vi "Check ref frame selected (simple).vi"() -> (3 "Proceed / Ref frame ok":bool)   [LabVIEW 2020]
uses:
  Typedefs/Set Main VI cursor.ctl
  Global Variables/General Globals.vi
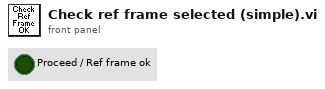
[diagram p1: front panel]
types:
  T1 = typedef "Set Main VI cursor.ctl" = enum16{"Release busy cursor", "Set busy cursor"}
  T2 = typedef "Reference_Globals.ctl" = cluster{"Refrence data path":path, "Reference Rectangle":i16[][], "AOL Z":dbl, "No of pixels in a miniscan ":i32[], "Threshold":i16[], "No of miniscans":i32[], "Full Frame Size":u16, "Reference Image":T3, "dwelltime":dbl, "Zoom":dbl, "Field of View":dbl, "Z Step":i8, "Z pixels":i32, "Z Lines":u8, "Z Ignore":u8, "Laser":u8}
  T3 = typedef "IMAQ Image.ctl" = refnum<image>
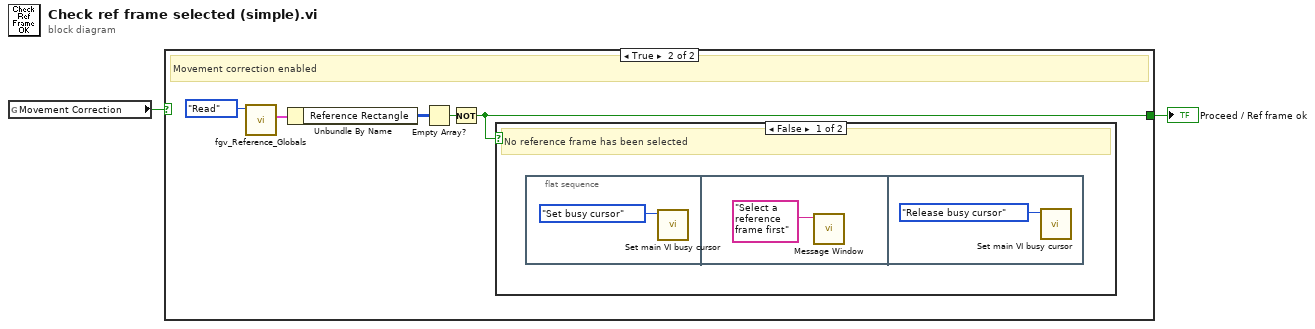
[diagram p0: block diagram]
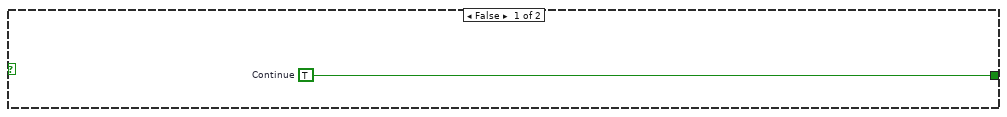
[diagram p2: hidden frame]
diagram:
  n1 = global read "General Globals.vi" "Movement Correction"() -> (w1:bool)
  n2 = case shown="True" w1 {
    tunnel: [w3 w4] -> w2
    frame False {
      w3 = TRUE  # Continue
    }
    frame True {
      # "Movement correction enabled"
      n3 = call "fgv_Reference_Globals.vi"("Function"=enum16{"Intialize", "Write", "Read", "Clear"}."Read") -> ("Reference Data"=w7:T2)  [unwired: 9 in, 1 out]
      n4 = Unbundle By Name(w7) -> ("Reference Rectangle"=w6:i16[][])
      n5 = Empty Array?(array=w6) -> (empty?=w5:bool)
      n6 = Not(x=w5) -> (.not. x?=w4:bool)
      n7 = case shown="False" w4 {
        frame False {
          # "No reference frame has been selected"
          n8 = flat-sequence {
            frame #0 {
              n9 = call "Set main VI busy cursor.vi"("Main VI's cursor"=Set_Main_VI_cursor."Set busy cursor") -> ()  [unwired: 10 in, 1 out]
            }
            frame #1 {
              n10 = call "Message Window.vi"("Message string"="Select a reference frame first") -> ()  [unwired: 10 in, 1 out]
            }
            frame #2 {
              n11 = call "Set main VI busy cursor.vi"("Main VI's cursor"=Set_Main_VI_cursor."Release busy cursor") -> ()  [unwired: 10 in, 1 out]
            }
          }
        }
        frame True {
          # "Reference frame has been selected"
        }
      }
    }
  }
  "Proceed / Ref frame ok" <- w2
